vi "draw.vi"(8 "error in (no error)":errorcluster, 11 "Circle in":refnum<class "Circle.lvclass">) -> (0 "error out":errorcluster, 3 "Circle out":refnum<class "Circle.lvclass">)   [LabVIEW 2018, in "Circle.lvclass"]
uses:
  Circle.lvclass
  Shape Class/Shape.lvclass
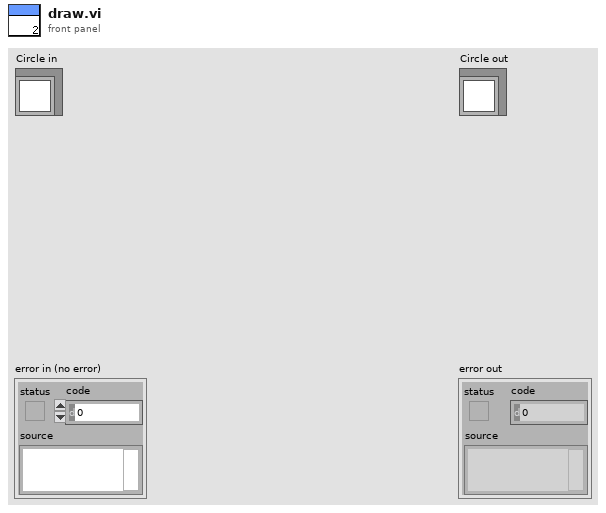
[diagram p1: front panel]
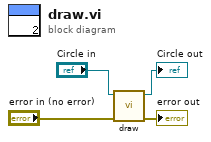
[diagram p0: block diagram]
diagram:
  n1 = call-parent "draw.vi"("error in (no error)"="error in (no error)", "Shape in"="Circle in") -> ("error out"=→"error out":errorcluster, "Shape out"=→"Circle out":refnum<class "Circle.lvclass">)  [unwired: 8 in]
